vi "TEST_bench_fgm_partial_pipeline_N22.vi"() -> ()   [LabVIEW 2017]
uses:
  fixed-point/single-axis/fxp_mpc/fgm_pipiline/quadProgParams_pipe.ctl
  <vilib>/rvi/Emulation/niFpgaEmulationIsFPGAContextNoSignature.vi
  <vilib>/rvi/DataTransferAndStorage/Container/Common/niFpgaContainerGetUniqueNameForEmu.vi
  <vilib>/rvi/Memory/Memory_Emulation/niFpgaMemoryEmulationCacheClearOnFirstRun.vi
  <vilib>/rvi/Memory/Memory_Emulation/nirvimemoryEmulationManagerCache_MakeExclusive.vi
  <vilib>/rvi/Memory/Memory_Emulation/niFpgaMemoryEmulationValidateCache.vi
  <vilib>/rvi/Memory/Memory_Emulation/nirvimemoryEmulationManagerCache_InsertValue.vi
  <vilib>/Utility/error.llb/Clear Errors.vi
  <vilib>/rvi/Memory/Memory_Emulation/nirvimemoryEmulationManagerCache_ReleaseExclusive.vi
  <vilib>/rvi/Memory/Memory_Emulation/nirvimemoryEmulationManagerCache_GetValue.vi
  <vilib>/rvi/Memory/Memory_Emulation/nirvimemoryEmulationManagerCache_SetValue.vi
  <vilib>/rvi/Emulation/niFpgaProcessEmulError.vi
  <vilib>/rvi/Emulation/niFpgaSctlEmulationGetInTimedLoop.vi
  <vilib>/rvi/Memory/Memory_Emulation/nirvimemoryFastEmulation.vi
  <vilib>/rvi/Memory/Memory_Emulation/nirvimemoryEmulation.vi
  <vilib>/rvi/errors/nirviReportUnexpectedCaseInternalError (U32).vi
  <vilib>/rvi/DataTransferAndStorage/Container/XNode/niFpgaContainer.xnode
  <vilib>/rvi/DataTransferAndStorage/Register/Emulation/niFpgaRegisterEmulation.vi
panel:
  out "z":fxp<+/-,32,6>[](array[numeric])
  out "y":fxp<+/-,32,6>[](array[numeric])
  in  "du_max":fxp<+/-,18,1>
  in  "QP_params":T1={"maxIter"=0, "nuN"=24, "Ns_mpc"=0, "-beta"=-0.9987945556640625, "beta+1"=1.9987945556640625}
  in  "idx2":i16=15
  in  "idx1":i16
  out "idx1":fxp<+/-,32,6>[](array[numeric])
  out "idx2":fxp<+/-,32,6>[](array[numeric])
  in  "z0":fxp<+/-,32,6>[](array[numeric])=[0.0, 0.0, 0.0, 0.0, 0.0, 0.0, 0.0, 0.0, 0.0, 0.0, 0.0, 0.0, 0.0, 0.0, 0.0, 0.0, 0.0, 0.0, 0.0, 0.0, 0.0, 0.0]
  in  "y0":fxp<+/-,32,6>[](array[numeric])=[0.0, 0.0, 0.0, 0.0, 0.0, 0.0, 0.0, 0.0, 0.0, 0.0, 0.0, 0.0, 0.0, 0.0, 0.0, 0.0, 0.0, 0.0, 0.0, 0.0, 0.0, 0.0]
  out "delta u(k)":fxp<+/-,32,3>
  in  "big_mat_data":fxp<+/-,32,3>[](array[numeric])=[0.0, 0.0, 0.0, 0.0, 0.0, 0.0, 0.0, 0.0, 0.0, 0.0, 0.0, 0.0]
  in  "x":fxp<+/-,32,6>[](array[numeric])=[0.0, 0.0, 0.0, 0.0, 0.0, 0.0, 0.0, 0.0, 0.0, 0.0, 0.0, 0.0, 0.0, 0.0, 0.0, 0.0, 0.0, 0.0, 0.0, 0.0, 0.0, 0.0, 0.0, 0.0, 0.0]
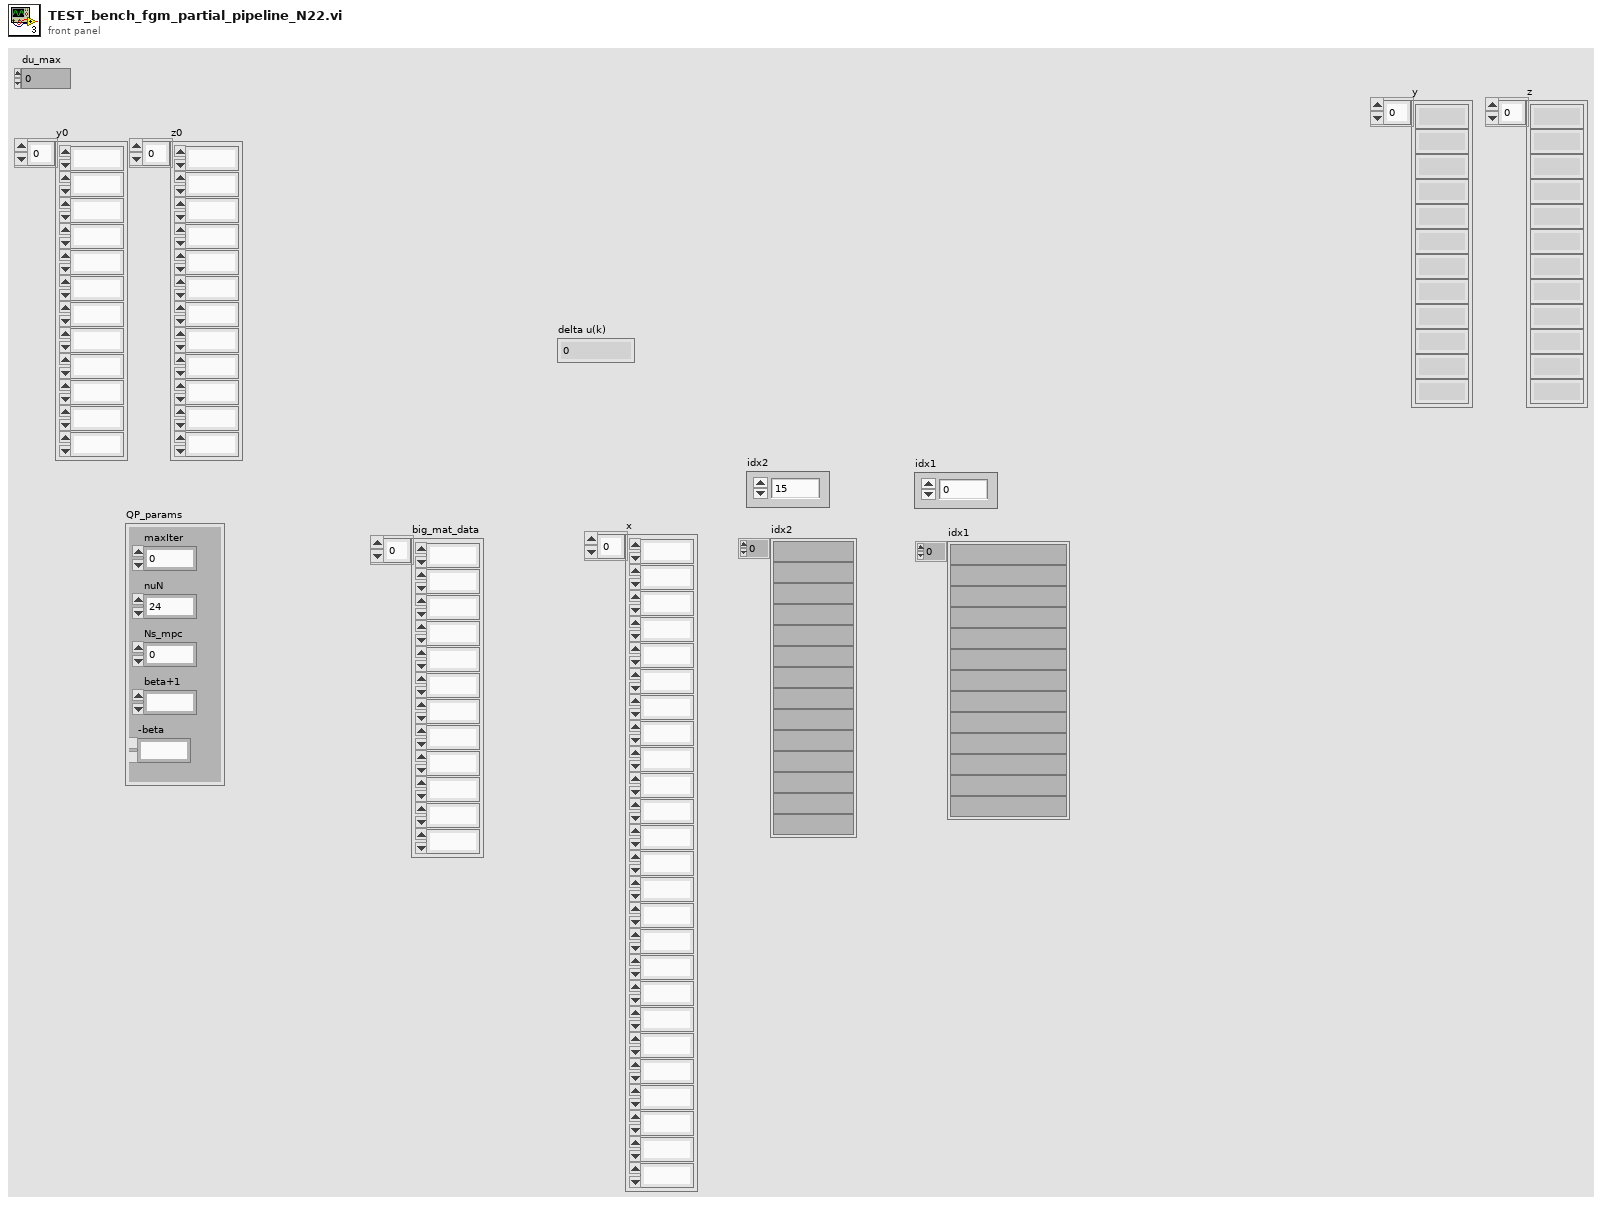
[diagram p1: front panel]
types:
  T1 = typedef "quadProgParams_pipe.ctl" = cluster{"maxIter":u16, "nuN":u16, "Ns_mpc":u16, "-beta":fxp<+/-,18,2>, "beta+1":fxp<+/-,18,2>}
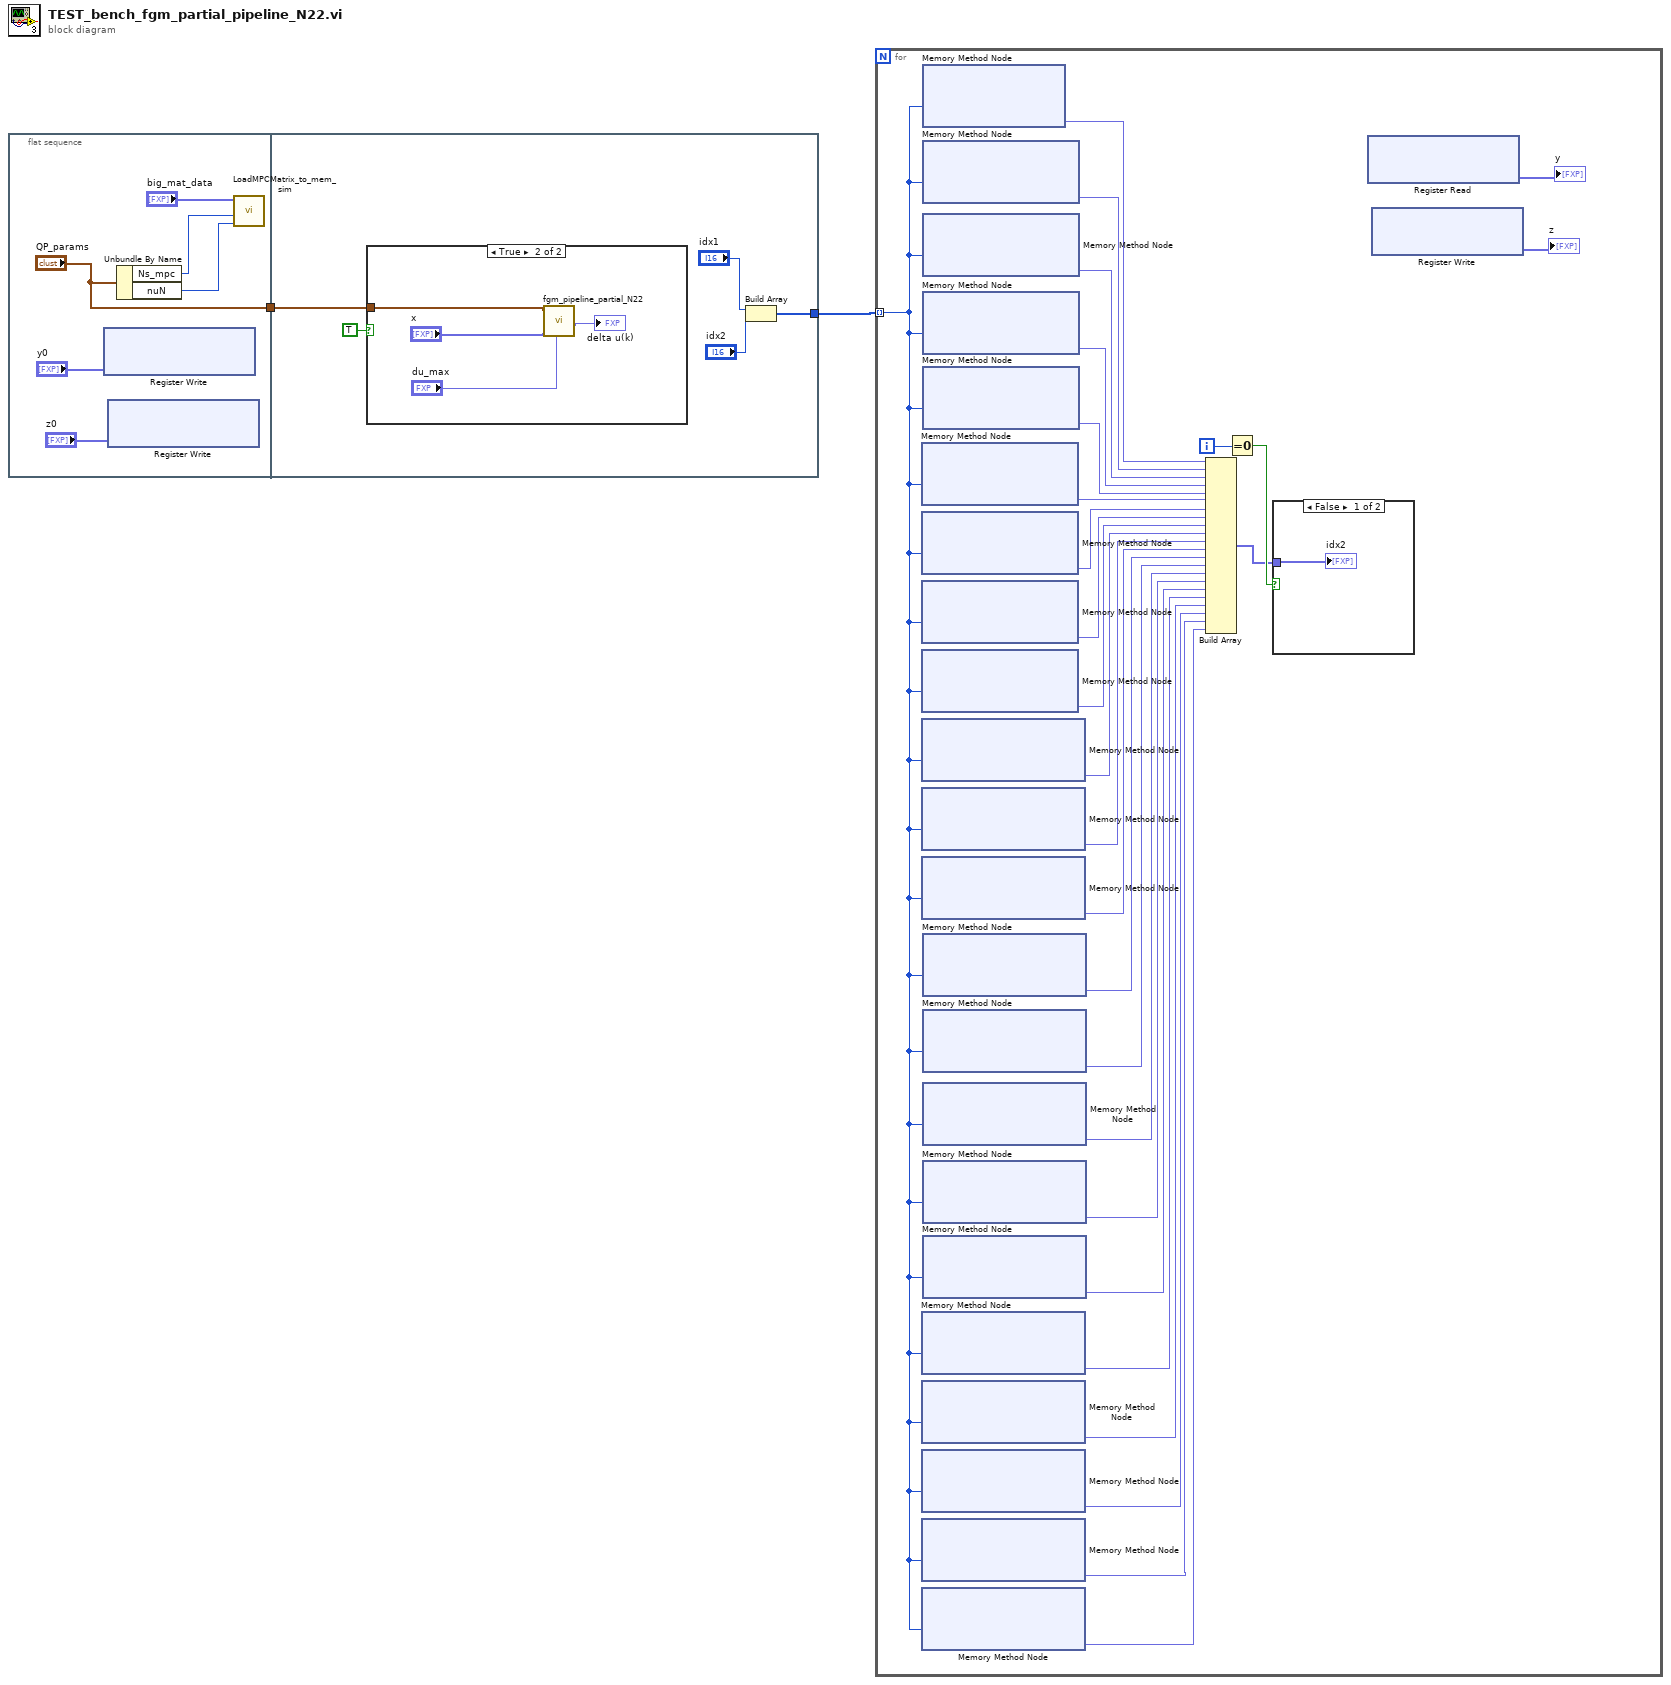
[diagram p0: block diagram]
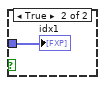
[diagram p2: hidden frame]
diagram:
  n1 = flat-sequence {
    tunnel: ["QP_params"] -> w2
    tunnel: [w13] -> w1
    tunnel: w2 -> [w12]
    frame #0 {
      n2 = xnode "Register Write"("Data"="y0") -> ()  [unwired: 1 in, 1 out]
      n3 = xnode "Register Write"("Data"="z0") -> ()  [unwired: 1 in, 1 out]
      n4 = Unbundle By Name("QP_params") -> ("Ns_mpc"=w6:u16, "nuN"=w7:u16)
      n5 = call "LoadMPCMatrix_to_mem_sim.vi"("nuN_mpc"=w7, "Ns"=w6, "big_mat_data"="big_mat_data") -> ()  [unwired: 9 in]
    }
    frame #1 {
      n6 = case shown="True" TRUE {
        tunnel: w12 -> [_ w17]
        frame False {
        }
        frame True {
          n7 = call "fgm_pipeline_partial_N22.vi"("du_max"="du_max", "x_vec"="x", "QP_params"=w17) -> ("delta u(k)"=→"delta u(k)":fxp<+/-,32,3>)  [unwired: 6 in, 2 out]
        }
      }
      n8 = Build Array("idx1", "idx2") -> (w13:i16[])
    }
  }
  n9 = for {
    tunnel: w1 -> [w21] mode=indexing
    i -> [w31]
    n10 = xnode ("Memory Method Node")("Address"=w21) -> ("Data"=w40:fxp<+/-,32,4>)  [unwired: 1 in, 1 out]
    n11 = xnode ("Memory Method Node")("Address"=w21) -> ("Data"=w39:fxp<+/-,32,4>)  [unwired: 1 in, 1 out]
    n12 = xnode ("Memory Method Node")("Address"=w21) -> ("Data"=w38:fxp<+/-,32,4>)  [unwired: 1 in, 1 out]
    n13 = xnode ("Memory Method Node")("Address"=w21) -> ("Data"=w37:fxp<+/-,32,4>)  [unwired: 1 in, 1 out]
    n14 = xnode ("Memory Method Node")("Address"=w21) -> ("Data"=w36:fxp<+/-,32,4>)  [unwired: 1 in, 1 out]
    n15 = xnode ("Memory Method Node")("Address"=w21) -> ("Data"=w35:fxp<+/-,32,4>)  [unwired: 1 in, 1 out]
    n16 = xnode ("Memory Method Node")("Address"=w21) -> ("Data"=w34:fxp<+/-,32,4>)  [unwired: 1 in, 1 out]
    n17 = xnode ("Memory Method Node")("Address"=w21) -> ("Data"=w25:fxp<+/-,32,4>)  [unwired: 1 in, 1 out]
    n18 = xnode ("Memory Method Node")("Address"=w21) -> ("Data"=w24:fxp<+/-,32,4>)  [unwired: 1 in, 1 out]
    n19 = xnode ("Memory Method Node")("Address"=w21) -> ("Data"=w23:fxp<+/-,32,4>)  [unwired: 1 in, 1 out]
    n20 = xnode ("Memory Method Node")("Address"=w21) -> ("Data"=w22:fxp<+/-,32,4>)  [unwired: 1 in, 1 out]
    n21 = xnode ("Memory Method Node")("Address"=w21) -> ("Data"=w20:fxp<+/-,32,4>)  [unwired: 1 in, 1 out]
    n22 = xnode ("Memory Method Node")("Address"=w21) -> ("Data"=w45:fxp<+/-,32,4>)  [unwired: 1 in, 1 out]
    n23 = xnode ("Memory Method Node")("Address"=w21) -> ("Data"=w44:fxp<+/-,32,4>)  [unwired: 1 in, 1 out]
    n24 = xnode ("Memory Method Node")("Address"=w21) -> ("Data"=w43:fxp<+/-,32,4>)  [unwired: 1 in, 1 out]
    n25 = xnode ("Memory Method Node")("Address"=w21) -> ("Data"=w42:fxp<+/-,32,4>)  [unwired: 1 in, 1 out]
    n26 = xnode ("Memory Method Node")("Address"=w21) -> ("Data"=w41:fxp<+/-,32,4>)  [unwired: 1 in, 1 out]
    n27 = xnode ("Memory Method Node")("Address"=w21) -> ("Data"=w30:fxp<+/-,32,4>)  [unwired: 1 in, 1 out]
    n28 = xnode ("Memory Method Node")("Address"=w21) -> ("Data"=w29:fxp<+/-,32,4>)  [unwired: 1 in, 1 out]
    n29 = xnode ("Memory Method Node")("Address"=w21) -> ("Data"=w28:fxp<+/-,32,4>)  [unwired: 1 in, 1 out]
    n30 = xnode ("Memory Method Node")("Address"=w21) -> ("Data"=w27:fxp<+/-,32,4>)  [unwired: 1 in, 1 out]
    n31 = xnode ("Memory Method Node")("Address"=w21) -> ("Data"=w26:fxp<+/-,32,4>)  [unwired: 1 in, 1 out]
    n32 = Build Array(w45, w44, w43, w42, w41, w40, w39, w38, w37, w36, w35, w34, w30, w29, w28, w27, w26, w25, w24, w23, w22, w20) -> (w32:fxp<+/-,32,4>[])
    n33 = Equal To 0?(x=w31) -> (x = 0?=w33:bool)
    n34 = case shown="False" w33 {
      tunnel: w32 -> [w46 w47]
      frame False {
        "idx2" <- w46
      }
      frame True {
        "idx1" <- w47
      }
    }
    n35 = xnode "Register Read"() -> ("Data"=→"y":fxp<+/-,32,6>[])  [unwired: 1 in, 1 out]
    n36 = xnode "Register Write"() -> ("Data"=→"z":fxp<+/-,32,6>[])  [unwired: 1 in, 1 out]
  }
